vi "SQL写入 - 穿管检测.vi"(0 "ADODB._Connection In":refnum<k7>, 5 "TestMessage":string, 11 "error in (no error)":errorcluster caption="错误输入（无错误）") -> (4 "ADODB._Connection Out":refnum<k7>, 15 "error out":errorcluster caption="错误输出")   [LabVIEW 2017]
panel:
  out "当前日期时间":string
  out "连接的字符串":string
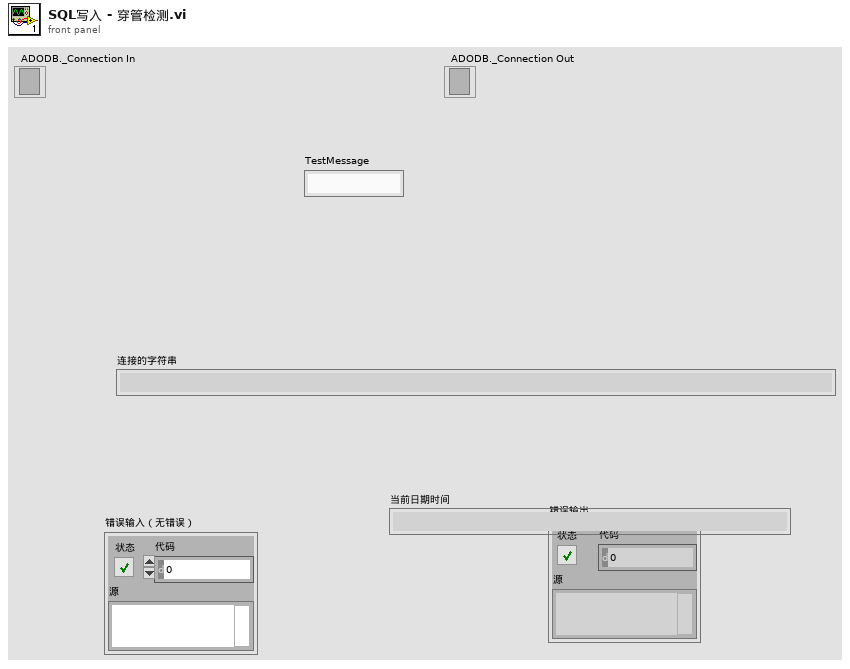
[diagram p1: front panel]
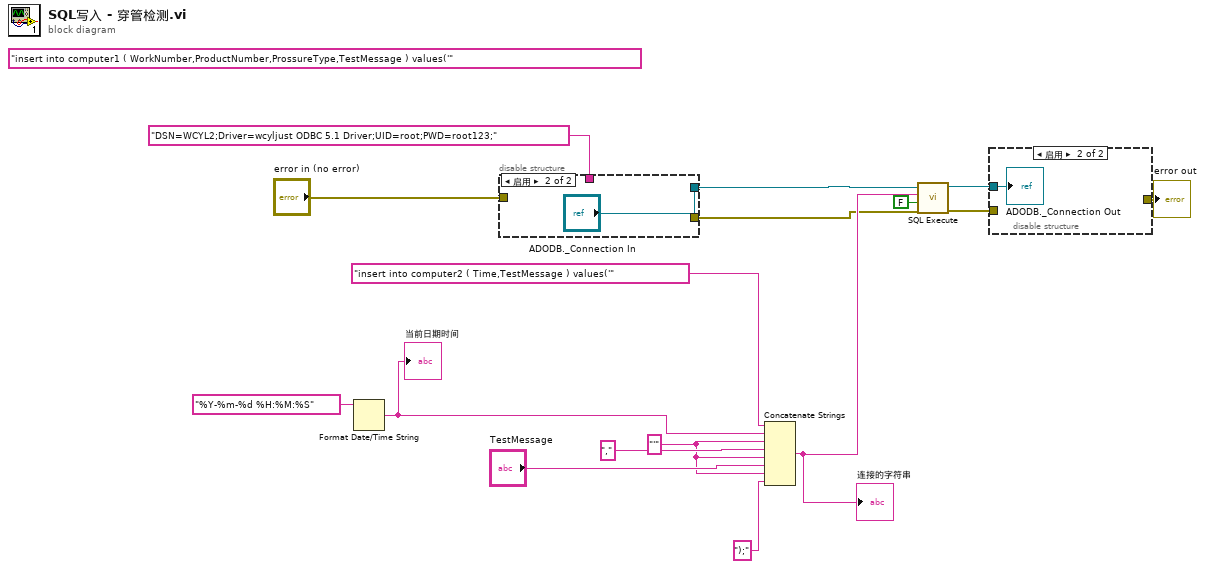
[diagram p0: block diagram]
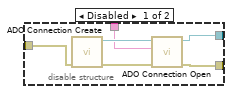
[diagram p2: hidden frame]
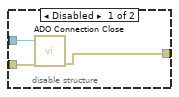
[diagram p3: hidden frame]
diagram:
  (unwired) "insert into computer1 ( WorkNumber,ProductNumber,ProssureType,TestMessage ) values('" ("Command Text")
  w13 = "'" ("字符串")
  n1 = Format Date/Time String(time format string (%c)="%Y-%m-%d %H:%M:%S" ("时间格式字符串(%c)")) -> (date/time string=w1:string)  [unwired: 2 in]
  "当前日期时间" <- w1
  n2 = disable-structure shown="启用" {
    disable-tunnel: "DSN=WCYL2;Driver=wcyljust ODBC 5.1 Driver;UID=root;PWD=root123;" ("ConnectionString") -> [w20 _]
    disable-tunnel: "error in (no error)" -> [w19 _]
    disable-tunnel: [w18 "ADODB._Connection In"] -> w5
    disable-tunnel: [w17 _] -> w4
    frame Disabled {
      n3 = call <userlib>:"ADO Connection Create.vi"("error in (no error)"=w19) -> ("error out"=w21:errorcluster, "ADODB._Connection Out"=w22:refnum<k7>)  [unwired: 9 in]
      n4 = call <userlib>:"ADO Connection Open.vi"("error in (no error)"=w21, "ConnectionString"=w20, "ADODB._Connection In"=w22) -> ("error out"=w17:errorcluster, "ADODB._Connection Out"=w18:refnum<k7>)  [unwired: 7 in]
    }
    frame Enabled {
    }
  }
  n5 = Concatenate Strings("insert into computer2 ( Time,TestMessage ) values('" ("Command Text"), w1, w13, "," ("字符串"), w13, "TestMessage", w13, ");" ("字符串")) -> (w11:string)
  "连接的字符串" <- w11
  n6 = call <userlib>:"SQL Execute.vi"("error in (no error)"=w4, "Return Data (T)"=FALSE, "Command Text"=w11, "ADODB._Connection In"=w5) -> ("error out"=w9:errorcluster, "ADODB._Connection Out"=w10:refnum<k7>)  [unwired: 4 in, 2 out]
  n7 = disable-structure shown="启用" {
    disable-tunnel: w10 -> [w26 w27]
    disable-tunnel: w9 -> [w25 _]
    disable-tunnel: [w24 _] -> w7
    frame Disabled {
      n8 = call <userlib>:"ADO Connection Close.vi"("error in (no error)"=w25, "ADODB._Connection In"=w26) -> ("error out"=w24:errorcluster)  [unwired: 8 in, 1 out]
    }
    frame Enabled {
      "ADODB._Connection Out" <- w27
    }
  }
  "error out" <- w7
